vi "Get Switch Names and Topology.vi"(8 "error in (no error)":errorcluster, 11 "CSV File":path=path "C:/Users/chericks/Desktop/P2_Module/P2_Module/Test Code/Test_Sense_Routes.csv") -> (0 "error out":errorcluster, 2 "Switch Topologies":T1[](array[typedef])=["2526/2-Wire 79x1 Mux", "2526/2-Wire 79x1 Mux", "2526/2-Wire 79x1 Mux", "Configured Topology", "Configured Topology", "Configured Topology", "Configured Topology", "Configured Topology", "Configured Topology", "Configured Topology", "Configured Topology", "Configured Topology", "Configured Topology", "Configured Topology", "Configured Topology", "Configured Topology", "Configured Topology", "Configured Topology", "Configured Topology", "Configured Topology"], 3 "Switch Resource Names":refnum<k15>[](array[refnum])=["2526_A", "2526_B", "2526_C", "2810_A1_SCSI1", "2810_A1_SCSI2", "2810_A1_SCSI3", "2810_A2_SCSI1", "2810_A2_SCSI2", "2810_A2_SCSI3", "2810_B1_SCSI1", "2810_B1_SCSI2", "2810_B1_SCSI3", "2810_B2_SCSI1", "2810_B2_SCSI2", "2810_B2_SCSI3", "2810_C1_SCSI1", "2810_C1_SCSI2", "2810_C2_SCSI1", "2810_C2_SCSI2", "2810_C2_SCSI3"])   [LabVIEW 2019]
uses:
  <instrlib>/niSwitch/niSwitch.llb/niSwitch Topologies.ctl
  3940470e-b812-4b81-afda-c7eceabf7a2f.vi
  <vilib>/Utility/file.llb/Read Delimited Spreadsheet (string).vi
panel:
  out "all rows":string[][](array[string])
  out "array with duplicates removed":string[](array[string])=["2526_A", "2526_B", "2526_C", "2810_A1_SCSI1", "2810_A1_SCSI2", "2810_A1_SCSI3", "2810_A2_SCSI1", "2810_A2_SCSI2", "2810_A2_SCSI3", "2810_B1_SCSI1", "2810_B1_SCSI2", "2810_B1_SCSI3", "2810_B2_SCSI1", "2810_B2_SCSI2", "2810_B2_SCSI3", "2810_C1_SCSI1", "2810_C1_SCSI2", "2810_C2_SCSI1", "2810_C2_SCSI2", "2810_C2_SCSI3"]
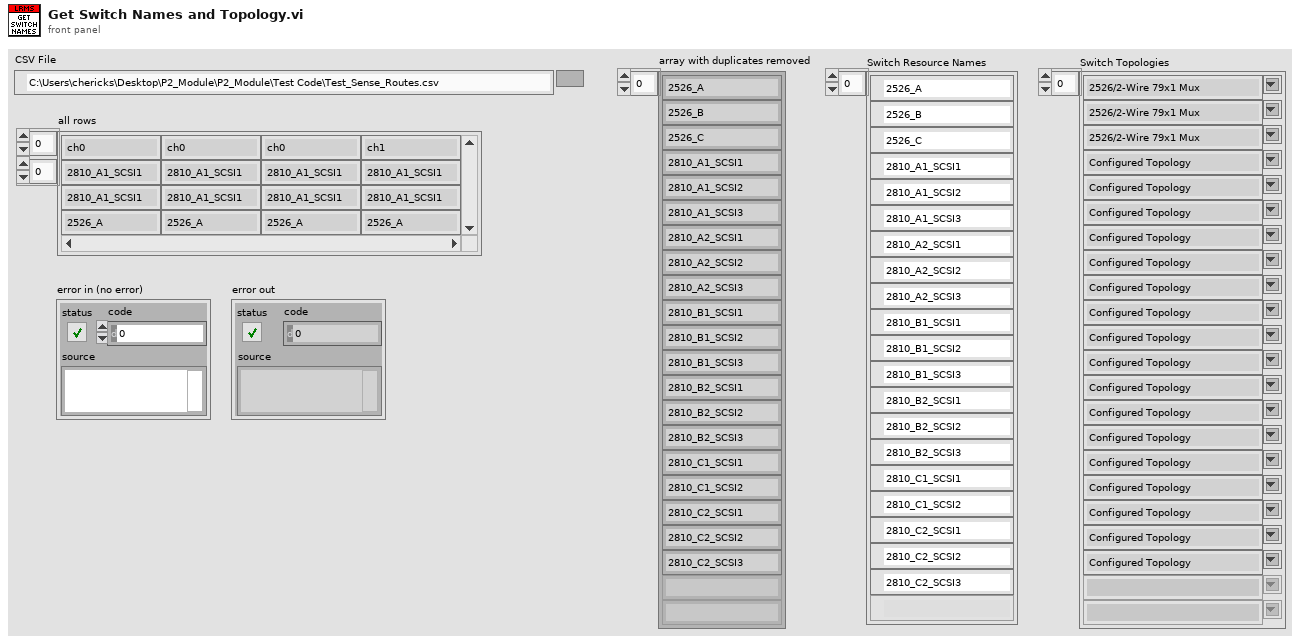
[diagram p1: front panel]
types:
  T1 = typedef "niSwitch Topologies.ctl" = string
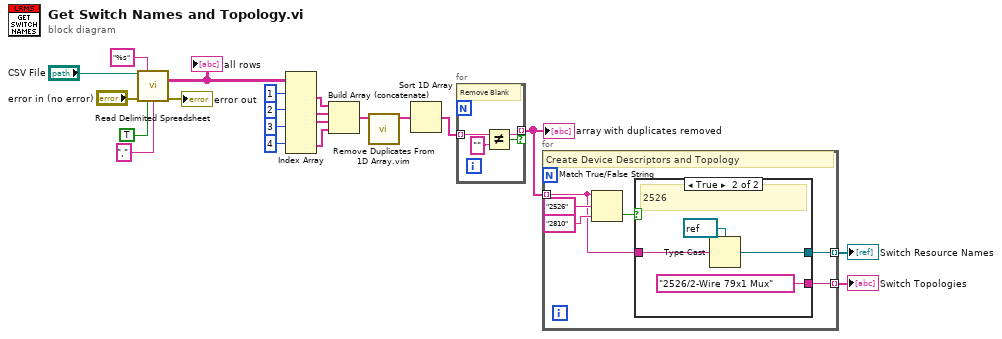
[diagram p0: block diagram]
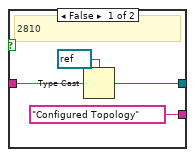
[diagram p2: hidden frame]
diagram:
  n1 = call-poly <vilib>:"Read Delimited Spreadsheet.vi"("file path (dialog if empty)"="CSV File", "format (%s)"="%s", "error in (no error)"="error in (no error)", "transpose? (F)"=TRUE ("transpose? (no:F)"), "delimiter (\\t)"=",") -> ("all rows"=w15:string[][], "error out"=→"error out":errorcluster)  [unwired: 5 in, 4 out]
  "all rows" <- w15
  n2 = Index Array(array=w15, index (row) #1=1 ("index (row)"), index (row) #2=2 ("index (row)"), index (row) #3=3 ("index (row)"), index (row) #4=4 ("index (row)")) -> (element #1=w9:string[], element #2=w8:string[], element #3=w7:string[], element #4=w6:string[])  [unwired: 4 in]
  n3 = Build Array (concatenate)(w9, w8, w7, w6) -> (w5:string[])
  n4 = call "Remove Duplicates From 1D Array.vim"("array"=w5) -> ("array with duplicates removed"=w10:string[])  [unwired: 10 in]
  n5 = Sort 1D Array(array=w10) -> (sorted array=w4:string[])
  n6 = for {
    tunnel: w4 -> [w23] mode=indexing
    tunnel: [w23] -> w3 mode=indexing if=w22
    # "Remove Blank"
    n7 = Not Equal?(x=w23, y="") -> (x != y?=w22:bool)
  }
  "array with duplicates removed" <- w3
  n8 = for {
    tunnel: w3 -> [w27] mode=indexing
    tunnel: [w26] -> w2 mode=indexing
    tunnel: [w25] -> w1 mode=indexing
    # "Create Device Descriptors and Topology"
    n9 = Match True/False String(2:"2810" ("false string"), 3:"2526" ("true string"), 4:w27) -> (0:w28:bool)  [unwired: 1 out]
    n10 = case shown="True" w28 {
      tunnel: w27 -> [w33 w37]
      tunnel: [w32 w36] -> w26
      tunnel: [T1 "Configured Topology" ("topology name") T1 "2526/2-Wire 79x1 Mux" ("topology name")] -> w25
      frame False {
        # "2810"
        n11 = Type Cast(type=refnum<k15> refnum ("resource name"), x=w33) -> (*(type *) &x=w32:refnum<k15>)
      }
      frame True {
        # "2526"
        n12 = Type Cast(type=refnum<k15> refnum ("resource name"), x=w37) -> (*(type *) &x=w36:refnum<k15>)
      }
    }
  }
  "Switch Resource Names" <- w2
  "Switch Topologies" <- w1
